vi "Main.vi"() -> ()   [LabVIEW 2022 SP3]
uses:
  <vilib>/Utility/miscctls.llb/LVRectTypeDef.ctl
  cb892d5d-d4df-4763-9c98-bc1f9a332ced.vi
  <vilib>/Instr/_visa.llb/VISA Configure Serial Port (Instr).vi
panel:
  out "connected?":bool
  in  "Device":refnum<visa-resource-name>
  in  "upload":bool
  in  "SO:":string
  in  "Operator:":string
  in  "Results":i32(listbox)
  in  "Stats":i32(listbox)
  in  "Tolerance(%)":string
  in  "Add":bool
  out "Read:":string
  in  "Evaulate":bool
  out "Result Box Plot":cluster{dbl[], dbl[]}[](graph)=[{[7.857142857142858, 2.142857142857143, 2.142857142857143, 7.857142857142858, 7.857142857142858, 2.142857142857143, 2.142857142857143], [20.0, 20.0, 0.75, 0.75, 54.75, 54.75, 20.0]}, {[], []}, {[5.0, 5.0, 5.0], [-100.0, 120.0, -80.0]}, {[5.0, 5.0], [54.75, 101.0]}, {[5.0, 5.0], [0.75, -61.0]}, {[6.428571428571429, 3.571428571428571], [101.0, 101.0]}, {[6.428571428571429, 3.571428571428571], [-61.0, -61.0]}, {[17.857142857142858, 12.142857142857142, 12.142857142857142, 17.857142857142858, 17.857142857142858, 12.142857142857142, 12.142857142857142], [8.5, 8.5, 1.5, 1.5, 38.5, 38.5, 8.5]}, {[], []}, {[15.0, 15.0], [100.0, -90.0]}, {[15.0, 15.0], [38.5, 64.0]}, {[15.0, 15.0], [1.5, -47.0]}, {[16.428571428571427, 13.571428571428571], [64.0, 64.0]}, {[16.428571428571427, 13.571428571428571], [-47.0, -47.0]}]
  in  "Clear":bool
  in  "Delete Row":bool
  out "Average":dbl
  out "Min":dbl
  out "Max":dbl
  in  "Target Weight":string
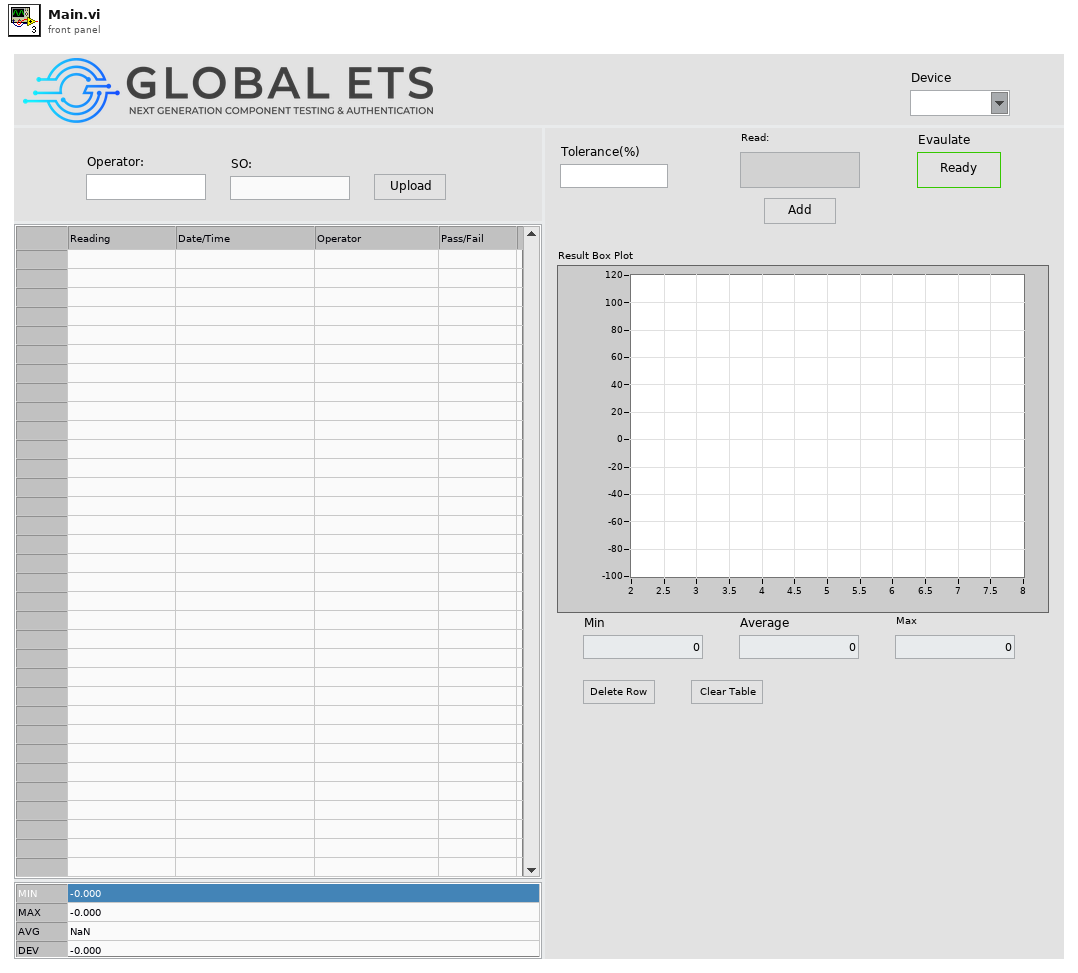
[diagram p1: front panel]
types:
  T1 = typedef "LVRowAndColumnTypeDef.ctl" = cluster{"Row":i32, "Column":i32}
  T2 = typedef "LVRectTypeDef.ctl" = cluster{"Left":i16, "Top":i16, "Right":i16, "Bottom":i16}
  T3 = typedef "imagedata.ctl" = cluster{"image type":i32, "image depth":i32, "image":u8[], "mask":u8[], "colors":u32[], "Rectangle":cluster{"left":i16, "top":i16, "right":i16, "bottom":i16}}
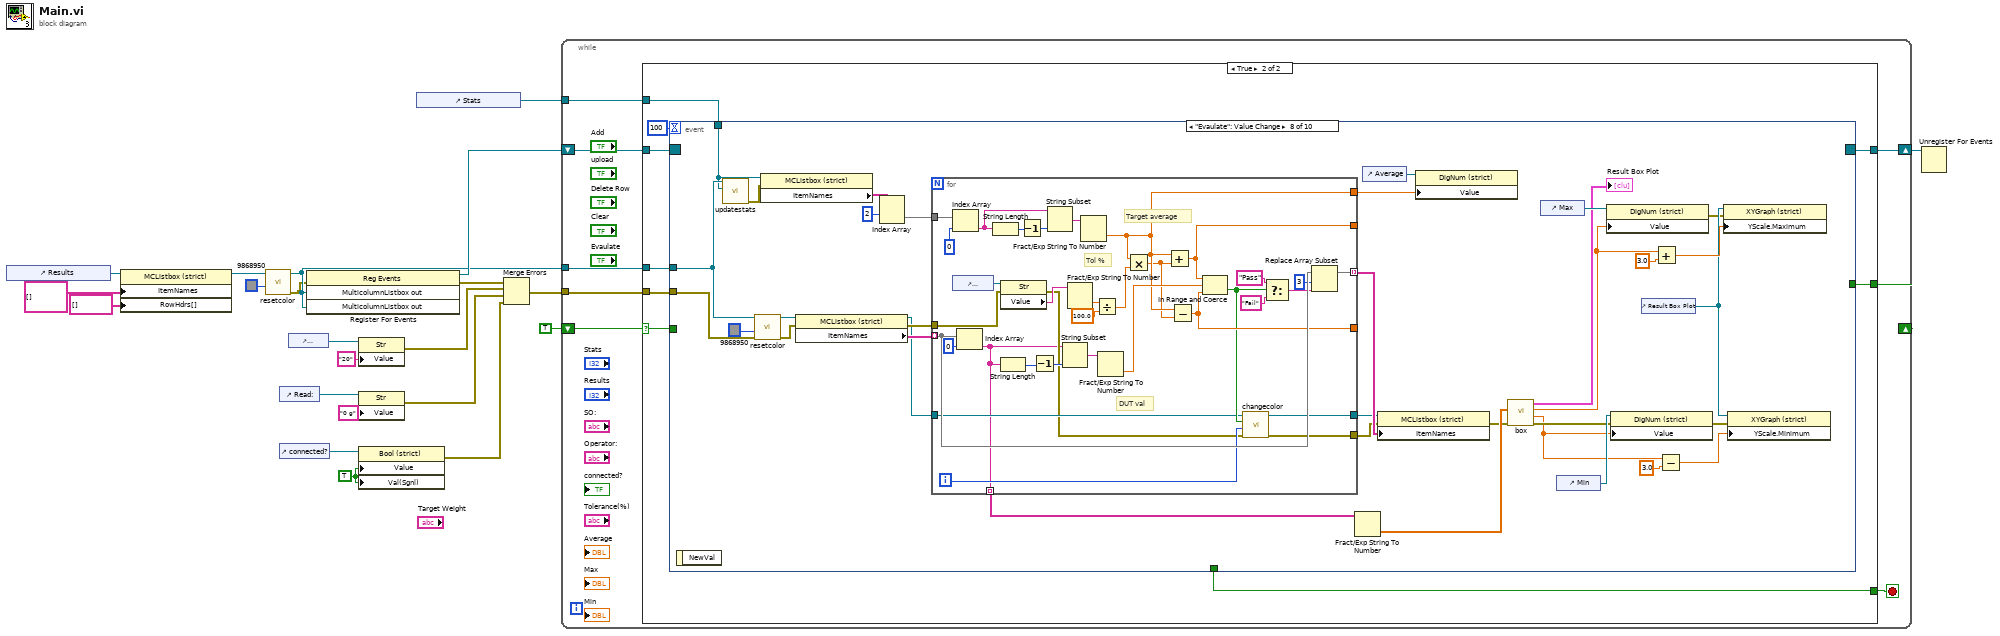
[diagram p0: block diagram]
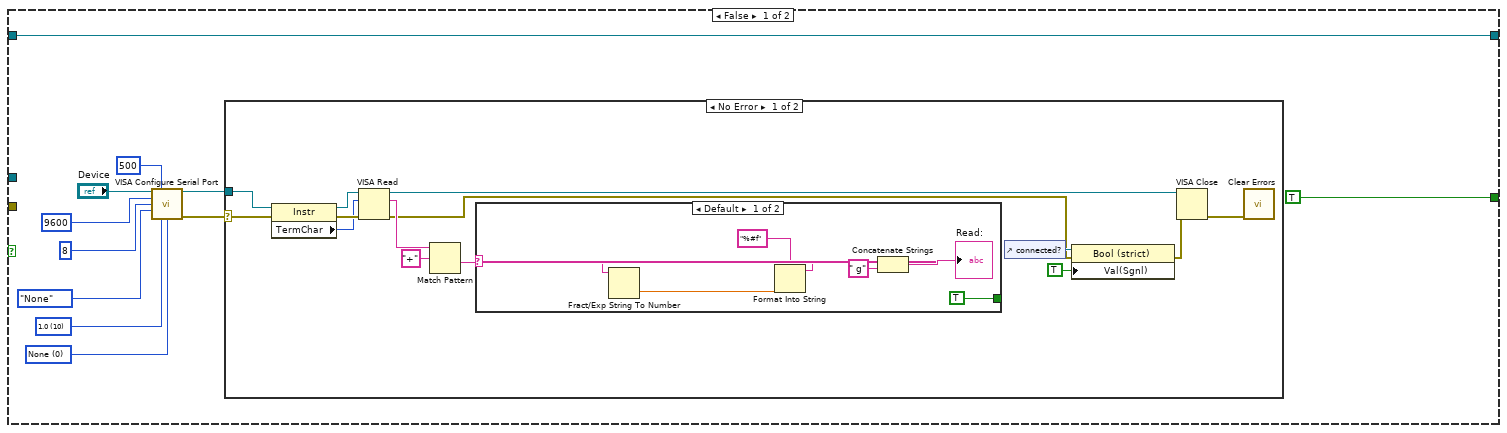
[diagram p2: hidden frame]
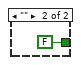
[diagram p3: hidden frame]
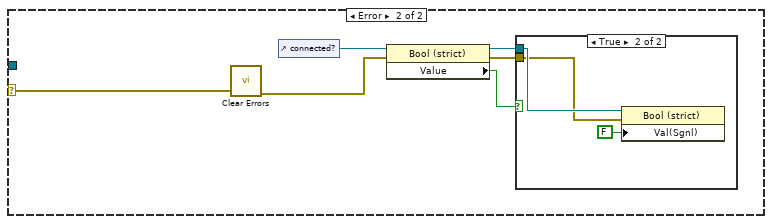
[diagram p4: hidden frame]
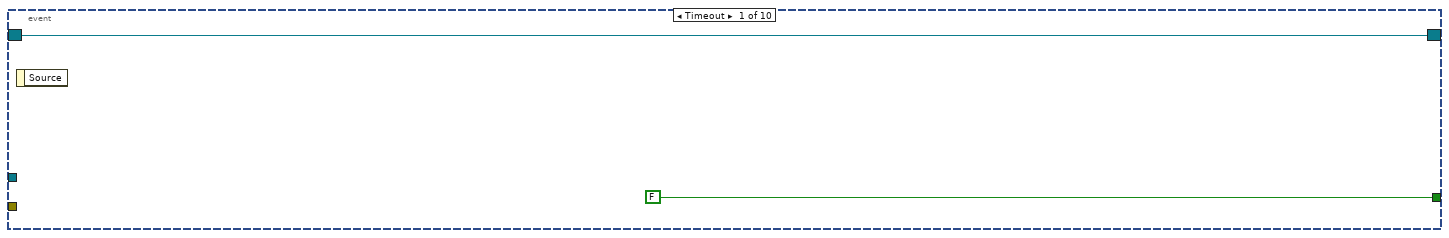
[diagram p6: hidden frame]
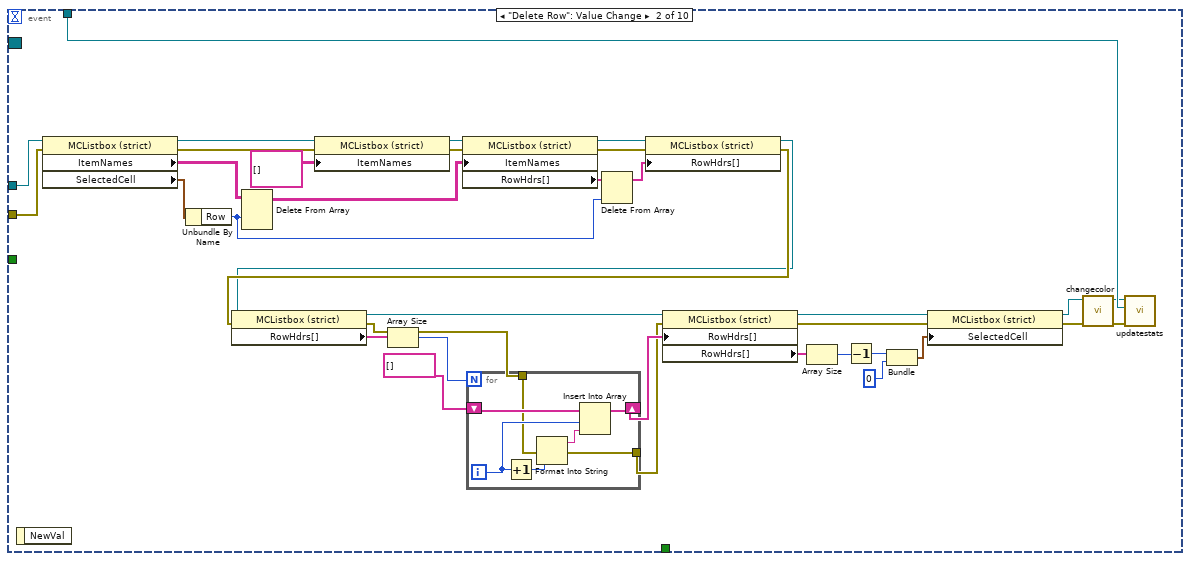
[diagram p7: hidden frame]
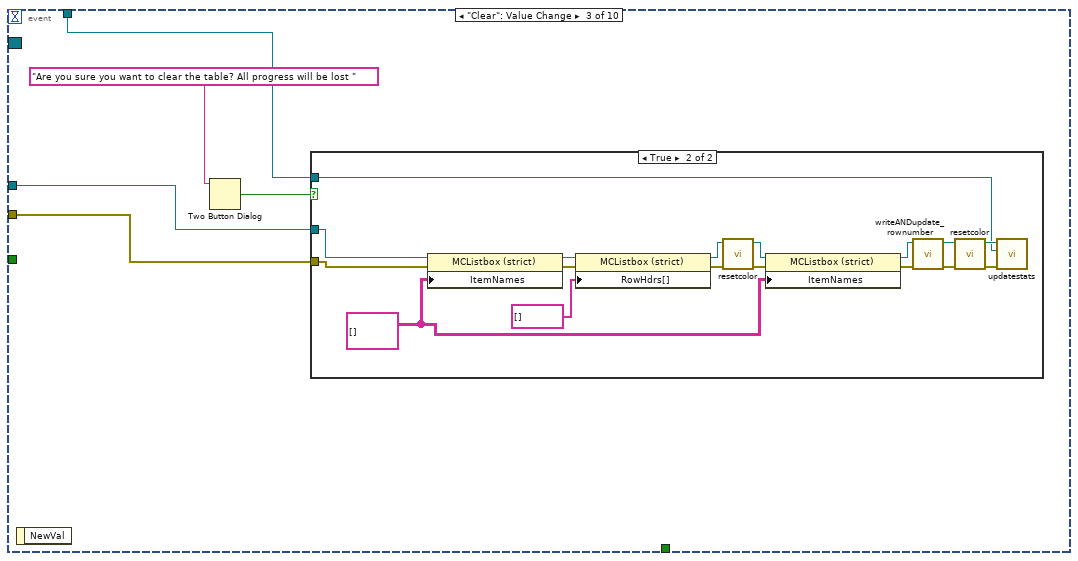
[diagram p8: hidden frame]
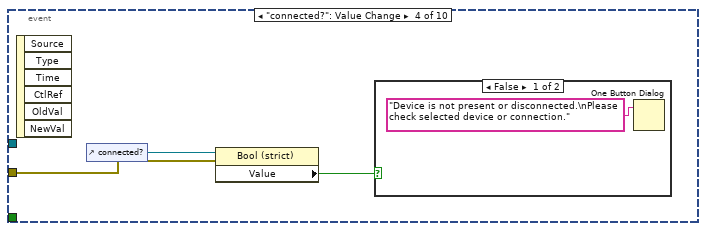
[diagram p10: hidden frame]
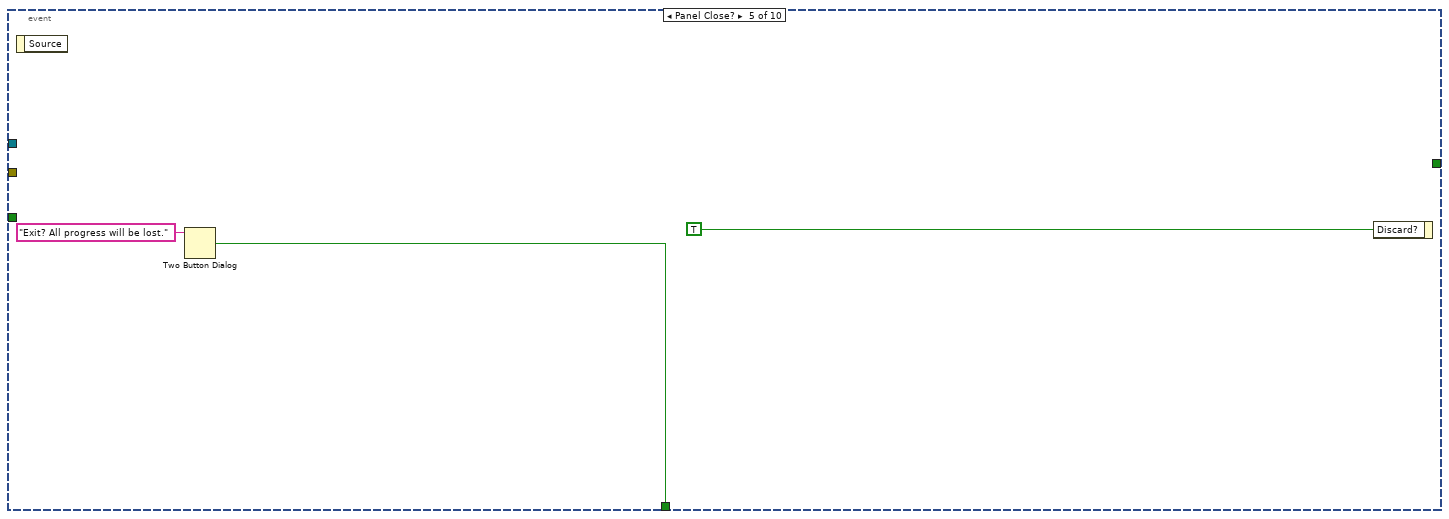
[diagram p12: hidden frame]
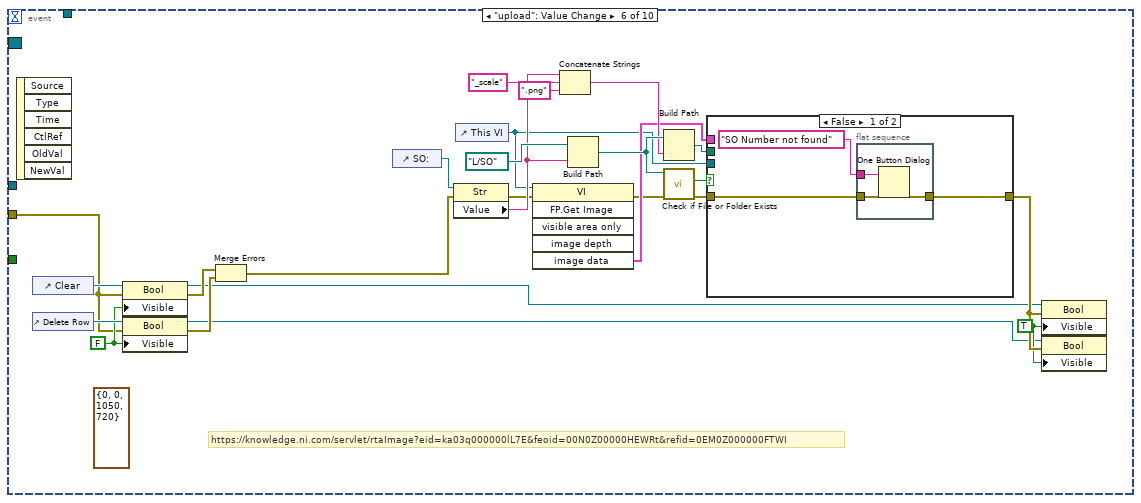
[diagram p13: hidden frame]
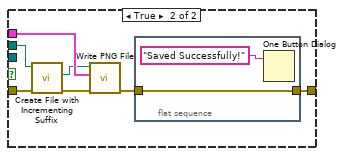
[diagram p14: hidden frame]
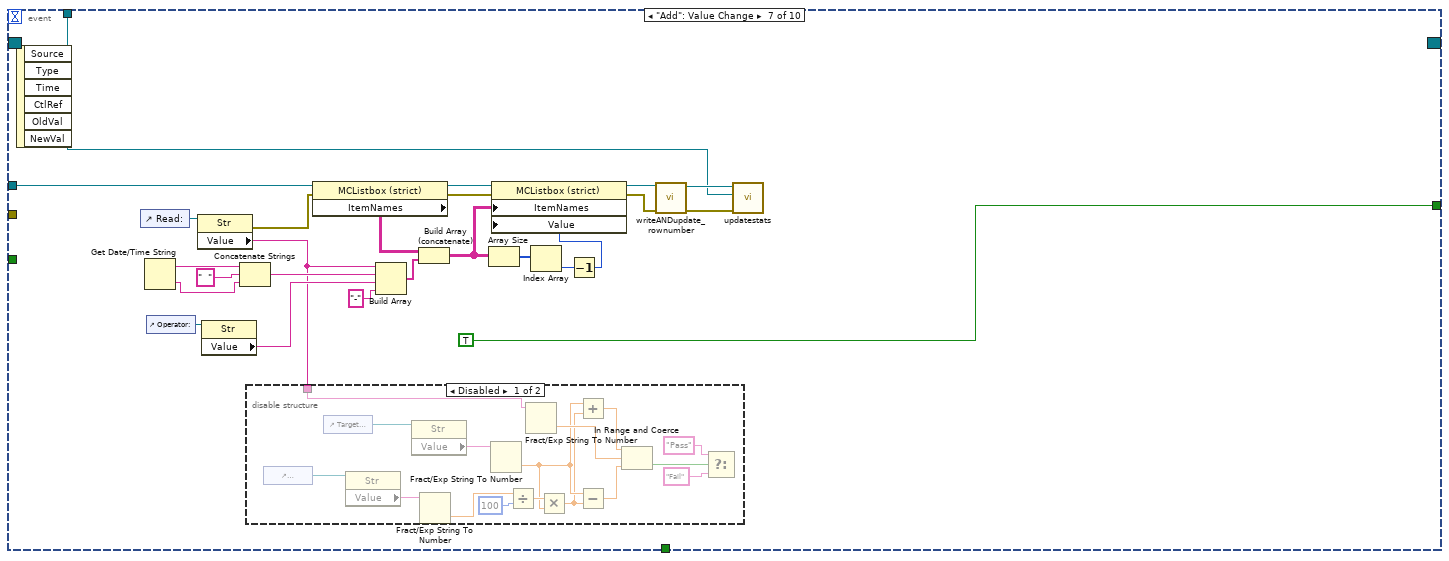
[diagram p15: hidden frame]
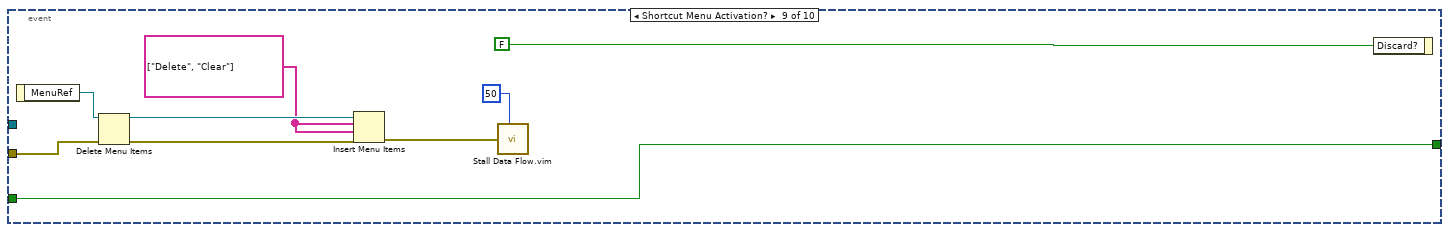
[diagram p17: hidden frame]
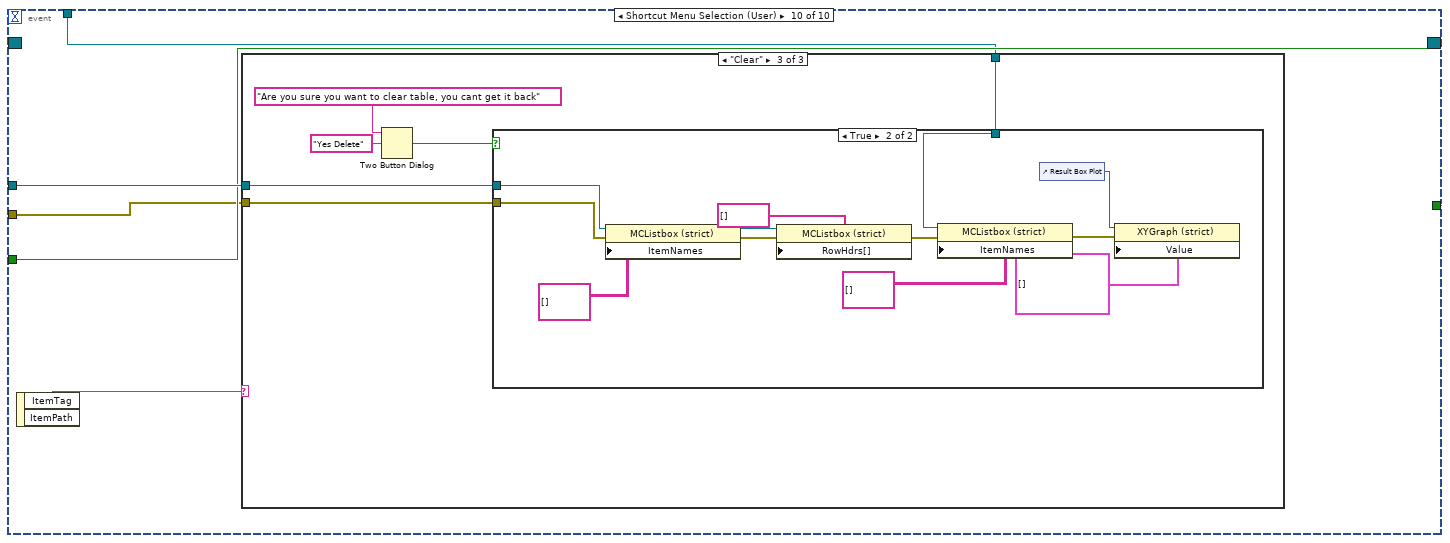
[diagram p18: hidden frame]
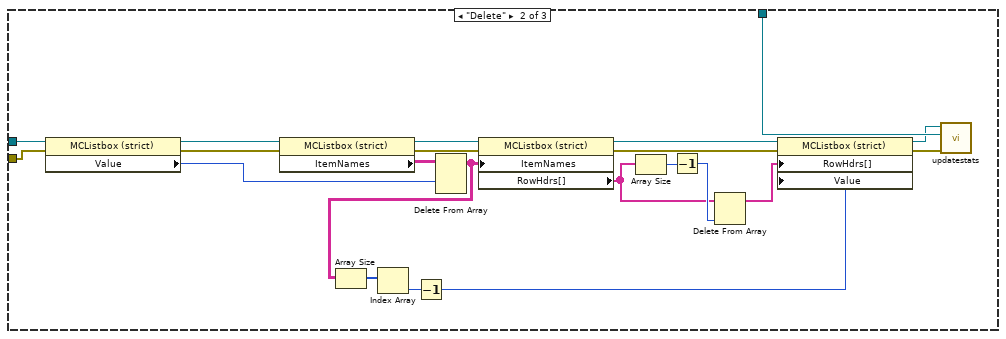
[diagram p20: hidden frame]
diagram:
  w7 = TRUE ("Value")
  n1 = control-ref of="Results"() -> (w14:refnum<vi>)
  n2 = property class="MCListbox (strict)"(reference=w14, "ItemNames"=string[][] [] ("Item Names"), "RowHdrs[]"=string[] [] ("Row Header Strings[]")) -> (reference out=w11:refnum<vi>)  [unwired: 1 in, 1 out]
  n3 = call "resetcolor.vi"("Color Box"=u32 9868950, "MulticolumnListbox in"=w11) -> ("error out"=w5:errorcluster, "MulticolumnListbox out"=w13:refnum<vi>)  [unwired: 8 in]
  n4 = control-ref of="Read:"() -> (w16:refnum<vi>)
  n5 = control-ref of="connected?"() -> (w8:refnum<vi>)
  n6 = control-ref of="Tolerance(%)"() -> (w17:refnum<vi>)
  n7 = register-events(error in=w5, w13, w13) -> (reference out=w19:refnum<event-registration>, error out=w20:errorcluster)  [unwired: 1 in]
  n8 = property class="Str"(reference=w17, "Value"="20") -> (error out=w3:errorcluster)  [unwired: 1 in, 1 out]
  n9 = property class="Str"(reference=w16, "Value"="0 g") -> (error out=w2:errorcluster)  [unwired: 1 in, 1 out]
  n10 = property class="Bool (strict)"(reference=w8, "Value"=w7, "Val(Sgnl)"=w7) -> (error out=w1:errorcluster)  [unwired: 1 in, 1 out]
  n11 = control-ref of="Stats"() -> (w6:refnum<vi>)
  n12 = Merge Errors(w20, w3, w2, w1) -> (w4:errorcluster)
  n13 = while {
    shift-right: [w29] -> _
    shift-left: TRUE -> [w30]
    tunnel: w13 -> [w27]
    tunnel: w4 -> [w26]
    shift-right: [w28] -> w21
    shift-left: w19 -> [w25]
    tunnel: w6 -> [w23]
    stop <- w24 stop-if-true
    n14 = case shown="True" w30 {
      selector: w30 -> [_ w75]
      tunnel: [TRUE w80] -> w29
      tunnel: w25 -> [w33 w79]
      tunnel: [w33 w78] -> w28
      tunnel: w27 -> [_ w77]
      tunnel: w26 -> [_ w76]
      tunnel: [_ w74] -> w24
      tunnel: w23 -> [_ w73]
      frame False {
        w35 = u16 0 items=["None", "XON/XOFF", "RTS/CTS", "XON/XOFF & RTS/CTS", "DTR/DSR", "XON/XOFF & DTR/DSR"] ("flow control (0:none)")
        w36 = u16 10 items=["1.0"=10, "1.5"=15, "2.0"=20] ("stop bits (10: 1 bit)")
        n15 = call-poly "VISA Configure Serial Port"("VISA resource name"="Device", "timeout (10sec)"=u32 500, "baud rate (9600)"=u32 9600, "data bits (8)"=u16 8, "parity (0:none)"=enum16{"None", "Odd", "Even", "Mark", "Space"}."None", "stop bits (10: 1 bit)"=w36, "flow control (0:none)"=w35) -> ("VISA resource name out"=w41:refnum<visa-resource-name>, "error out"=w32:errorcluster)  [unwired: 7 in]
        n16 = case shown="No Error" w32 {
          selector: w32 -> [w46 w69]
          tunnel: w41 -> [w55 _]
          frame No Error {
            n17 = property class="Instr"(reference=w55, error in=w46) -> (reference out=w51:refnum<visa-resource-name>, error out=w52:errorcluster, "TermChar"=w50:u8)
            n18 = VISA Read(VISA resource name=w51, byte count=w50, error in (no error)=w52) -> (VISA resource name out=w54:refnum<visa-resource-name>, read buffer=w49:string, error out=w44:errorcluster)  [unwired: 1 out]
            n19 = Match Pattern(string=w49, regular expression="+") -> (after substring=w47:string)  [unwired: 1 in, 3 out]
            n20 = case shown="Default" w47 {
              selector: w47 -> [w61 _]
              tunnel: [TRUE FALSE] -> _
              frame Default {
                n21 = Fract/Exp String To Number(string=w61) -> (number=w60:dbl)  [unwired: 3 in, 1 out]
                n22 = Format Into String(format string="%#f", w60) -> (resulting string=w59:string)  [unwired: 2 in, 1 out]
                n23 = Concatenate Strings(w59, " g" ("string")) -> (→"Read:":string)
              }
              frame "" {
              }
            }
            n24 = control-ref of="connected?"() -> (w45:refnum<vi>)
            n25 = property class="Bool (strict)"(reference=w45, error in=w44, "Val(Sgnl)"=TRUE ("Value")) -> (error out=w43:errorcluster)  [unwired: 1 out]
            n26 = VISA Close(VISA resource name=w54, error in (no error)=w43) -> (error out=w53:errorcluster)
            n27 = call <vilib>:"Clear Errors.vi"("error in (no error)"=w53) -> ()  [unwired: 5 in, 2 out]
          }
          frame Error {
            n28 = call <vilib>:"Clear Errors.vi"("error in (no error)"=w69) -> ("error out"=w66:errorcluster)  [unwired: 5 in, 1 out]
            n29 = control-ref of="connected?"() -> (w68:refnum<vi>)
            n30 = property class="Bool (strict)"(reference=w68, error in=w66) -> (reference out=w67:refnum<vi>, error out=w65:errorcluster, "Value"=w64:bool)
            n31 = case shown="True" w64 {
              tunnel: w67 -> [_ w71]
              tunnel: w65 -> [_ w70]
              frame False {
              }
              frame True {
                n32 = property class="Bool (strict)"(reference=w71, error in=w70, "Val(Sgnl)"=FALSE ("Value")) -> ()  [unwired: 2 out]
              }
            }
          }
        }
      }
      frame True {
        n33 = event shown="[7] \"Evaulate\": Value Change" {
          selector: w79 -> [w83 _ _ _ _ _ _ _ _ _]
          dyn-events: [w83 _ _ _ _ _ _ _ _ _] -> w78
          timeout: 100 -> [_ _ _ _ _ _ _ _ _ _]
          tunnel: [FALSE _ _ _ _ _ TRUE _ w305 w315] -> w80
          tunnel: w77 -> [_ w87 w128 _ _ _ w209 w239 _ w316]
          tunnel: w76 -> [_ w97 w129 w149 _ w163 _ w254 w306 w313]
          tunnel: w75 -> [_ _ _ _ _ _ _ _ w305 w315]
          tunnel: [_ _ _ _ w154 _ _ _ _ _] -> w74
          tunnel: w73 -> [_ w88 w127 _ _ _ w201 w237 _ w314]
          event Timeout {
            n34 = event-data() -> ()  [unwired: 1 in, 1 out]
          }
          event "Delete Row": Value Change {
            n35 = event-data() -> ()  [unwired: 1 in, 1 out]
            n36 = property on="Property Node" class="MCListbox (strict)"(reference=w87, error in=w97) -> (reference out=w114:refnum<vi>, error out=w118:errorcluster, "ItemNames"=w119:string[][], "SelectedCell"=w98:T1)
            n37 = Unbundle By Name(w98) -> ("Row"=w111:i32)
            n38 = Delete From Array(array=w119, index (row)=w111) -> (array with subset deleted=w115:string[][])  [unwired: 2 in, 1 out]
            n39 = property on="Property Node" class="MCListbox (strict)"(reference=w114, error in=w118, "ItemNames"=string[][] [] ("Item Names")) -> (reference out=w113:refnum<vi>, error out=w116:errorcluster)
            n40 = property on="Property Node" class="MCListbox (strict)"(reference=w113, error in=w116, "ItemNames"=w115) -> (reference out=w110:refnum<vi>, error out=w109:errorcluster, "RowHdrs[]"=w85:string[])
            n41 = Delete From Array(array=w85, index=w111) -> (array with subset deleted=w112:string[])  [unwired: 1 in, 1 out]
            n42 = property on="Property Node" class="MCListbox (strict)"(reference=w110, error in=w109, "RowHdrs[]"=w112) -> (reference out=w96:refnum<vi>, error out=w108:errorcluster)
            n43 = property class="MCListbox (strict)"(reference=w96, error in=w108) -> (reference out=w90:refnum<vi>, error out=w95:errorcluster, "RowHdrs[]"=w107:string[])
            n44 = Array Size(array=w107) -> (size(s)=w94:i32)
            n45 = for {
              N: w94 -> [_]
              shift-right: [w126] -> w93
              shift-left: string[] [] ("Row Header Strings[]") -> [w124]
              tunnel: [w121] -> w92
              tunnel: w95 -> [w120]
              i -> [w125]
              n46 = Increment(x=w125) -> (x+1=w123:i32)
              n47 = Format Into String(error in=w120, w123) -> (resulting string=w122:string, error out=w121:errorcluster)  [unwired: 2 in]
              n48 = Insert Into Array(array=w124, index=w125, new element=w122) -> (w126:string[])
            }
            n49 = property class="MCListbox (strict)"(reference=w90, error in=w92, "RowHdrs[]"=w93) -> (reference out=w101:refnum<vi>, error out=w102:errorcluster, "RowHdrs[]"=w84:string[])
            n50 = Array Size(array=w84) -> (size(s)=w104:i32)
            n51 = Decrement(x=w104) -> (x-1=w103:i32)
            n52 = Bundle(w103, "Number of Rows"=u32 0) -> (w105:cluster{i32, "Number of Rows":u32})  [unwired: 1 in]
            n53 = property class="MCListbox (strict)"(reference=w101, error in=w102, "SelectedCell"=w105) -> (reference out=w99:refnum<vi>, error out=w100:errorcluster)
            n54 = call "changecolor.vi"("error in (no error)"=w100, "MulticolumnListbox in"=w99) -> ("error out"=w89:errorcluster, "MulticolumnListbox out"=w86:refnum<vi>)  [unwired: 8 in]
            n55 = call "updatestats.vi"("error in (no error)"=w89, "Stats Ref"=w88, "Result Ref"=w86) -> ()  [unwired: 7 in, 2 out]
          }
          event "Clear": Value Change {
            n56 = event-data() -> ()  [unwired: 1 in, 1 out]
            n57 = Two Button Dialog(message="Are you sure you want to clear the table? All progress will be lost ") -> (T button?=w130:bool)  [unwired: 2 in]
            n58 = case shown="True" w130 {
              tunnel: w129 -> [_ w138]
              tunnel: w128 -> [_ w137]
              tunnel: w127 -> [_ w133]
              frame False {
              }
              frame True {
                w142 = string[][] [] ("Item Names")
                n59 = property class="MCListbox (strict)"(reference=w137, error in=w138, "ItemNames"=w142) -> (reference out=w147:refnum<vi>, error out=w148:errorcluster)
                n60 = property class="MCListbox (strict)"(reference=w147, error in=w148, "RowHdrs[]"=string[] [] ("Row Header Strings[]")) -> (reference out=w139:refnum<vi>, error out=w140:errorcluster)
                n61 = call "resetcolor.vi"("error in (no error)"=w140, "MulticolumnListbox in"=w139) -> ("error out"=w141:errorcluster, "MulticolumnListbox out"=w136:refnum<vi>)  [unwired: 8 in]
                n62 = property class="MCListbox (strict)"(reference=w136, error in=w141, "ItemNames"=w142) -> (reference out=w144:refnum<vi>, error out=w145:errorcluster)
                n63 = call "writeANDupdate_rownumber.vi"("error in (no error)"=w145, "reference"=w144) -> ("error out"=w135:errorcluster, "reference out"=w143:refnum<vi>)  [unwired: 8 in]
                n64 = call "resetcolor.vi"("error in (no error)"=w135, "MulticolumnListbox in"=w143) -> ("error out"=w132:errorcluster, "MulticolumnListbox out"=w134:refnum<vi>)  [unwired: 8 in]
                n65 = call "updatestats.vi"("error in (no error)"=w132, "Stats Ref"=w133, "Result Ref"=w134) -> ()  [unwired: 7 in, 2 out]
              }
            }
          }
          event "connected?": Value Change {
            n66 = event-data() -> ()  [unwired: 1 in, 6 out]
            n67 = control-ref of="connected?"() -> (w151:refnum<vi>)
            n68 = property class="Bool (strict)"(reference=w151, error in=w149) -> ("Value"=w150:bool)  [unwired: 2 out]
            n69 = case shown="False" w150 {
              frame False {
                n70 = One Button Dialog(message="Device is not present or disconnected.\nPlease check selected device or connection.") -> ()  [unwired: 1 in, 1 out]
              }
              frame True {
              }
            }
          }
          event Panel Close? {
            n71 = event-data() -> ()  [unwired: 1 in, 1 out]
            n72 = Two Button Dialog(message="Exit? All progress will be lost.") -> (T button?=w154:bool)  [unwired: 2 in]
            n73 = event-data("Discard?"=TRUE) -> ()  [unwired: 1 in, 1 out]
          }
          event "upload": Value Change {
            w158 = TRUE ("Visible")
            w164 = FALSE ("Visible")
            (unwired) T2 {"Left"=0, "Top"=0, "Right"=1050, "Bottom"=720} ("Front Panel Window:Window Bounds")
            # "https://knowledge.ni.com/servlet/rtaImage?eid=ka03q000000lL7E&feoid=00N0Z00000HEWRt&refid=0EM0Z000000FTWI"
            n74 = event-data() -> ()  [unwired: 1 in, 6 out]
            n75 = control-ref of="Clear"() -> (w166:refnum<vi>)
            n76 = control-ref of="Delete Row"() -> (w165:refnum<vi>)
            n77 = property class="Bool"(reference=w166, error in=w163, "Visible"=w164) -> (reference out=w157:refnum<vi>, error out=w162:errorcluster)
            n78 = property class="Bool"(reference=w165, error in=w163, "Visible"=w164) -> (reference out=w156:refnum<vi>, error out=w160:errorcluster)
            n79 = Merge Errors(w162, w160) -> (w161:errorcluster)
            n80 = control-ref of="SO:"() -> (w180:refnum<vi>)
            n81 = property class="Str"(reference=w180, error in=w161) -> (error out=w171:errorcluster, "Value"=w176:string)  [unwired: 1 out]
            n82 = control-ref of="This VI"() -> (w168:refnum<vi>)
            n83 = invoke class="VI" method="FP.Get Image"(reference=w168, error in=w171) -> (error out=w170:errorcluster, "image data"=w172:T3)  [unwired: 4 in, 4 out]
            n84 = Concatenate Strings(w176, "_scale" ("string"), ".png" ("string")) -> (w174:string)
            n85 = Build Path(base path=path "L:/SO", name or relative path=w176) -> (appended path=w177:path)
            n86 = Build Path(base path=w177, name or relative path=w174) -> (appended path=w173:path)
            n87 = call <vilib>:"Check if File or Folder Exists.vi"("error in (no error)"=w170, "path"=w177) -> ("error out"=w169:errorcluster, "file or folder exists?"=w178:bool)  [unwired: 7 in, 1 out]
            n88 = case shown="False" w178 {
              tunnel: w173 -> [_ w189]
              tunnel: w172 -> [_ w192]
              tunnel: w169 -> [w183 w191]
              tunnel: [w181 w190] -> w159
              tunnel: w168 -> [_ _]
              frame False {
                n89 = flat-sequence {
                  tunnel: "SO Number not found" ("message") -> [w185]
                  tunnel: w183 -> [w184]
                  tunnel: [w184] -> w181
                  frame #0 {
                    n90 = One Button Dialog(message=w185) -> ()  [unwired: 1 in, 1 out]
                  }
                }
              }
              frame True {
                n91 = call <vilib>:"Create File with Incrementing Suffix.vi"("error in (no error)"=w191, "file path"=w189) -> ("error out"=w187:errorcluster, "actual path"=w188:path)  [unwired: 7 in, 1 out]
                n92 = call <vilib>:"Write PNG File.vi"("error in (no error)"=w187, "image data"=w192, "path to PNG file"=w188) -> ("error out"=w186:errorcluster)  [unwired: 7 in, 1 out]
                n93 = flat-sequence {
                  tunnel: w186 -> [w193]
                  tunnel: [w193] -> w190
                  frame #0 {
                    n94 = One Button Dialog(message="Saved Successfully!") -> ()  [unwired: 1 in, 1 out]
                  }
                }
              }
            }
            n95 = property class="Bool"(reference=w157, error in=w159, "Visible"=w158) -> ()  [unwired: 2 out]
            n96 = property class="Bool"(reference=w156, error in=w159, "Visible"=w158) -> ()  [unwired: 2 out]
          }
          event "Add": Value Change {
            n97 = event-data() -> ()  [unwired: 1 in, 6 out]
            n98 = control-ref of="Read:"() -> (w219:refnum<vi>)
            n99 = Get Date/Time String() -> (date string=w208:string, time string=w206:string)  [unwired: 3 in]
            n100 = control-ref of="Operator:"() -> (w218:refnum<vi>)
            n101 = property class="Str"(reference=w219) -> (error out=w214:errorcluster, "Value"=w202:string)  [unwired: 1 in, 1 out]
            n102 = property class="Str"(reference=w218) -> ("Value"=w210:string)  [unwired: 1 in, 2 out]
            n103 = Concatenate Strings(w208, "  " ("string"), w206) -> (w211:string)
            n104 = disable-structure shown="Disabled" {
              disable-tunnel: w202 -> [w228 _]
              frame Disabled {
                n105 = control-ref of="Tolerance(%)"() -> (w235:refnum<vi>)
                n106 = control-ref of="Target Weight"() -> (w234:refnum<vi>)
                n107 = property class="Str"(reference=w235) -> ("Value"=w231:string)  [unwired: 1 in, 2 out]
                n108 = property class="Str"(reference=w234) -> ("Value"=w229:string)  [unwired: 1 in, 2 out]
                n109 = Fract/Exp String To Number(string=w231) -> (number=w230:dbl)  [unwired: 3 in, 1 out]
                n110 = Fract/Exp String To Number(string=w229) -> (number=w221:dbl)  [unwired: 3 in, 1 out]
                n111 = Divide(x=w230, y=100) -> (x/y=w232:dbl)
                n112 = Fract/Exp String To Number(string=w228) -> (number=w227:dbl)  [unwired: 3 in, 1 out]
                n113 = Multiply(x=w232, y=w221) -> (x*y=w220:dbl)
                n114 = Add(x=w221, y=w220) -> (x+y=w226:dbl)
                n115 = Subtract(x=w221, y=w220) -> (x-y=w225:dbl)
                n116 = In Range and Coerce(upper limit=w226, x=w227, lower limit=w225) -> (In Range?=w224:bool)  [unwired: 1 out]
                n117 = Select(t="Pass" ("Value"), s=w224, f="Fail" ("Value")) -> ()  [unwired: 1 out]
              }
              frame Enabled {
              }
            }
            n118 = property class="MCListbox (strict)"(reference=w209, error in=w214) -> (reference out=w213:refnum<vi>, error out=w215:errorcluster, "ItemNames"=w217:string[][])
            n119 = Build Array(w202, w211, w210, "-" ("element")) -> (w216:string[])
            n120 = Build Array (concatenate)(w217, w216) -> (w198:string[][])
            n121 = Array Size(array=w198) -> (size(s)=w197:i32[])
            n122 = Index Array(array=w197) -> (element=w196:i32)  [unwired: 1 in]
            n123 = Decrement(x=w196) -> (x-1=w195:i32)
            n124 = property class="MCListbox (strict)"(reference=w213, error in=w215, "ItemNames"=w198, "Value"=w195) -> (reference out=w199:refnum<vi>, error out=w205:errorcluster)
            n125 = call "writeANDupdate_rownumber.vi"("error in (no error)"=w205, "reference"=w199) -> ("error out"=w204:errorcluster, "reference out"=w203:refnum<vi>)  [unwired: 8 in]
            n126 = call "updatestats.vi"("error in (no error)"=w204, "Stats Ref"=w201, "Result Ref"=w203) -> ()  [unwired: 7 in, 2 out]
          }
          event "Evaulate": Value Change {
            n127 = event-data() -> ()  [unwired: 1 in, 1 out]
            n128 = call "updatestats.vi"("Stats Ref"=w237, "Result Ref"=w239) -> ("error IO"=w238:errorcluster)  [unwired: 8 in, 1 out]
            n129 = call "resetcolor.vi"("error in (no error)"=w254, "Color Box"=u32 9868950, "MulticolumnListbox in"=w239) -> ("error out"=w255:errorcluster, "MulticolumnListbox out"=w256:refnum<vi>)  [unwired: 7 in]
            n130 = property class="MCListbox (strict)"(reference=w237, error in=w238) -> ("ItemNames"=w269:string[][])  [unwired: 2 out]
            n131 = property class="MCListbox (strict)"(reference=w256, error in=w255) -> (reference out=w259:refnum<vi>, error out=w265:errorcluster, "ItemNames"=w267:string[][])
            n132 = Index Array(array=w269, index (row)=2) -> (element=w268:string[])  [unwired: 1 in]
            n133 = for {
              tunnel: w268 -> [w271]
              tunnel: w267 -> [w299] mode=indexing
              tunnel: [w296] -> w266 mode=indexing
              tunnel: w265 -> [w274]
              tunnel: [w275] -> w264
              tunnel: [w289] -> _
              tunnel: [w288] -> _
              tunnel: [w281] -> w260
              tunnel: w259 -> [w276]
              tunnel: [w278] -> w258
              tunnel: [w272] -> w252 mode=indexing
              i -> [w277]
              # "DUT val"
              # "Tol %"
              # "Target average"
              n134 = Index Array(array=w271, index=0) -> (element=w270:string)
              n135 = control-ref of="Tolerance(%)"() -> (w284:refnum<vi>)
              n136 = Index Array(array=w299, index=0 ("index (row)")) -> (element=w272:string)
              n137 = String Length(string=w270) -> (length=w295:i32)
              n138 = String Length(string=w272) -> (length=w291:i32)
              n139 = property class="Str"(reference=w284, error in=w274) -> (error out=w273:errorcluster, "Value"=w286:string)  [unwired: 1 out]
              n140 = Decrement(x=w295) -> (x-1=w294:i32)
              n141 = Decrement(x=w291) -> (x-1=w292:i32)
              n142 = String Subset(string=w270, length (rest)=w294) -> (substring=w293:string)  [unwired: 1 in]
              n143 = String Subset(string=w272, length (rest)=w292) -> (substring=w290:string)  [unwired: 1 in]
              n144 = Fract/Exp String To Number(string=w286) -> (number=w285:dbl)  [unwired: 3 in, 1 out]
              n145 = Fract/Exp String To Number(string=w293) -> (number=w281:dbl)  [unwired: 3 in, 1 out]
              n146 = Divide(x=w285, y=100.0) -> (x/y=w282:dbl)
              n147 = Fract/Exp String To Number(string=w290) -> (number=w287:dbl)  [unwired: 3 in, 1 out]
              n148 = Multiply(x=w281, y=w282) -> (x*y=w280:dbl)
              n149 = Add(x=w281, y=w280) -> (x+y=w289:dbl)
              n150 = Subtract(x=w281, y=w280) -> (x-y=w288:dbl)
              n151 = In Range and Coerce(upper limit=w289, x=w287, lower limit=w288) -> (In Range?=w279:bool)  [unwired: 1 out]
              n152 = call "changecolor.vi"("error in (no error)"=w273, "Numeric"=w277, "Boolean"=w279, "MulticolumnListbox in"=w276) -> ("error out"=w275:errorcluster, "MulticolumnListbox out"=w278:refnum<vi>)  [unwired: 6 in]
              n153 = Select(t="Pass" ("Value"), s=w279, f="Fail" ("Value")) -> (s? t:f=w297:string)
              n154 = Replace Array Subset(array=w299, new element=w297, index=3) -> (w296:string[])
            }
            n155 = Fract/Exp String To Number(string=w252) -> (number=w253:dbl[])  [unwired: 3 in, 1 out]
            n156 = control-ref of="Average"() -> (w263:refnum<vi>)
            n157 = property class="MCListbox (strict)"(reference=w258, error in=w264, "ItemNames"=w266) -> (error out=w246:errorcluster)  [unwired: 1 out]
            n158 = property class="DigNum (strict)"(reference=w263, "Value"=w260) -> ()  [unwired: 1 in, 2 out]
            n159 = call "box.vi"("error in (no error)"=w246, "Plot 1 Data"=w253) -> ("error out"=w244:errorcluster, "min"=w243:dbl, "max"=w242:dbl, "Box Plot"=→"Result Box Plot":cluster{dbl[], dbl[]}[])  [unwired: 6 in]
            n160 = control-ref of="Max"() -> (w261:refnum<vi>)
            n161 = control-ref of="Min"() -> (w262:refnum<vi>)
            n162 = property class="DigNum (strict)"(reference=w261, "Value"=w242) -> (error out=w240:errorcluster)  [unwired: 1 in, 1 out]
            n163 = property class="DigNum (strict)"(reference=w262, error in=w244, "Value"=w243) -> (error out=w251:errorcluster)  [unwired: 1 out]
            n164 = control-ref of="Result Box Plot"() -> (w241:refnum<vi>)
            n165 = Add(x=w242, y=3.0) -> (x+y=w247:dbl)
            n166 = Subtract(x=w243, y=3.0) -> (x-y=w249:dbl)
            n167 = property class="XYGraph (strict)"(reference=w241, error in=w240, "YScale.Maximum"=w247) -> ()  [unwired: 2 out]
            n168 = property class="XYGraph (strict)"(reference=w241, error in=w251, "YScale.Minimum"=w249) -> ()  [unwired: 2 out]
          }
          event Shortcut Menu Activation? {
            w309 = string[] ["Delete", "Clear"] ("item names")
            n169 = event-data() -> ("MenuRef"=w312:refnum<k9>)  [unwired: 1 in]
            n170 = Delete Menu Items(6:w306, 9:w312) -> (0:w311:errorcluster, 3:w310:refnum<k9>)  [unwired: 2 in]
            n171 = Insert Menu Items(6:w311, 7:w309, 8:w309, 9:w310) -> (0:w308:errorcluster)  [unwired: 2 in, 2 out]
            n172 = call "Stall Data Flow.vim"("value in"=w308, "milliseconds to wait"=u32 50) -> ()  [unwired: 2 out]
            n173 = event-data("Discard?"=FALSE) -> ()  [unwired: 1 in, 1 out]
          }
          event Shortcut Menu Selection (User) {
            n174 = event-data() -> ("ItemTag"=w317:string)  [unwired: 1 in, 1 out]
            n175 = case shown="\"Clear\"" w317 {
              tunnel: w316 -> [_ w336 w341]
              tunnel: w314 -> [_ w337 w340]
              tunnel: w313 -> [_ w322 w339]
              frame Default {
              }
              frame "Delete" {
                n176 = property class="MCListbox (strict)"(reference=w336, error in=w322) -> (reference out=w332:refnum<vi>, error out=w324:errorcluster, "Value"=w334:i32)
                n177 = property class="MCListbox (strict)"(reference=w332, error in=w324) -> (reference out=w331:refnum<vi>, error out=w325:errorcluster, "ItemNames"=w333:string[][])
                n178 = Delete From Array(array=w333, index (row)=w334) -> (array with subset deleted=w319:string[][])  [unwired: 2 in, 1 out]
                n179 = Array Size(array=w319) -> (size(s)=w321:i32[])
                n180 = Index Array(array=w321) -> (element=w320:i32)  [unwired: 1 in]
                n181 = Decrement(x=w320) -> (x-1=w318:i32)
                n182 = property class="MCListbox (strict)"(reference=w331, error in=w325, "ItemNames"=w319) -> (reference out=w329:refnum<vi>, error out=w328:errorcluster, "RowHdrs[]"=w323:string[])
                n183 = Array Size(array=w323) -> (size(s)=w330:i32)
                n184 = Decrement(x=w330) -> (x-1=w327:i32)
                n185 = Delete From Array(array=w323, index=w327) -> (array with subset deleted=w326:string[])  [unwired: 1 in, 1 out]
                n186 = property class="MCListbox (strict)"(reference=w329, error in=w328, "RowHdrs[]"=w326, "Value"=w318) -> (reference out=w335:refnum<vi>, error out=w338:errorcluster)
                n187 = call "updatestats.vi"("error in (no error)"=w338, "Stats Ref"=w337, "Result Ref"=w335) -> ()  [unwired: 7 in, 2 out]
              }
              frame "Clear" {
                n188 = Two Button Dialog(message="Are you sure you want to clear table, you cant get it back", 2:"Yes Delete" ("T button name (\"OK\")")) -> (T button?=w342:bool)  [unwired: 1 in]
                n189 = case shown="True" w342 {
                  tunnel: w341 -> [_ w355]
                  tunnel: w340 -> [_ w350]
                  tunnel: w339 -> [_ w346]
                  frame False {
                  }
                  frame True {
                    n190 = property class="MCListbox (strict)"(reference=w355, error in=w346, "ItemNames"=string[][] [] ("Item Names")) -> (reference out=w354:refnum<vi>, error out=w353:errorcluster)
                    n191 = property class="MCListbox (strict)"(reference=w354, error in=w353, "RowHdrs[]"=string[] [] ("Row Header Strings[]")) -> (error out=w351:errorcluster)  [unwired: 1 out]
                    n192 = property class="MCListbox (strict)"(reference=w350, error in=w351, "ItemNames"=string[][] [] ("Item Names")) -> (error out=w347:errorcluster)  [unwired: 1 out]
                    n193 = control-ref of="Result Box Plot"() -> (w345:refnum<vi>)
                    n194 = property class="XYGraph (strict)"(reference=w345, error in=w347, "Value"=cluster{dbl[], dbl[]}[] []) -> ()  [unwired: 2 out]
                  }
                }
              }
            }
          }
        }
      }
    }
  }
  n195 = Unregister For Events(event registration refnum=w21) -> ()  [unwired: 1 in, 1 out]
